vi "map_trap_piastre_stiffback.vi"() -> ()   [LabVIEW 2015]
panel:
  out "Mapping file":string
  in  "Done ?":bool
  in  "KILL":bool
  in  "PAUSE":bool
  in  "RESUME":bool
  in  "QUIT":bool
  in  "Done":bool
  in  "z piastra":bool
  in  "x piastra":bool
  in  "goto y pos":bool
  in  "goto x pos":bool
  in  "End":bool
  in  "zero z - end":bool
  in  "zero x - end":bool
  in  "zero y - end":bool
  in  "positioning done":bool
  out "output":string
  out "command":string
  in  "zero done":bool
  in  "zero z":bool
  in  "zero x":bool
  in  "zero y":bool
  # "Comandi di emergenza"
  # "Posiziono in zero"
  # "Vado sulla piastra \ne azzero"
  # "Vado in posizione\ne parto"
  # "Ritorno a zero"
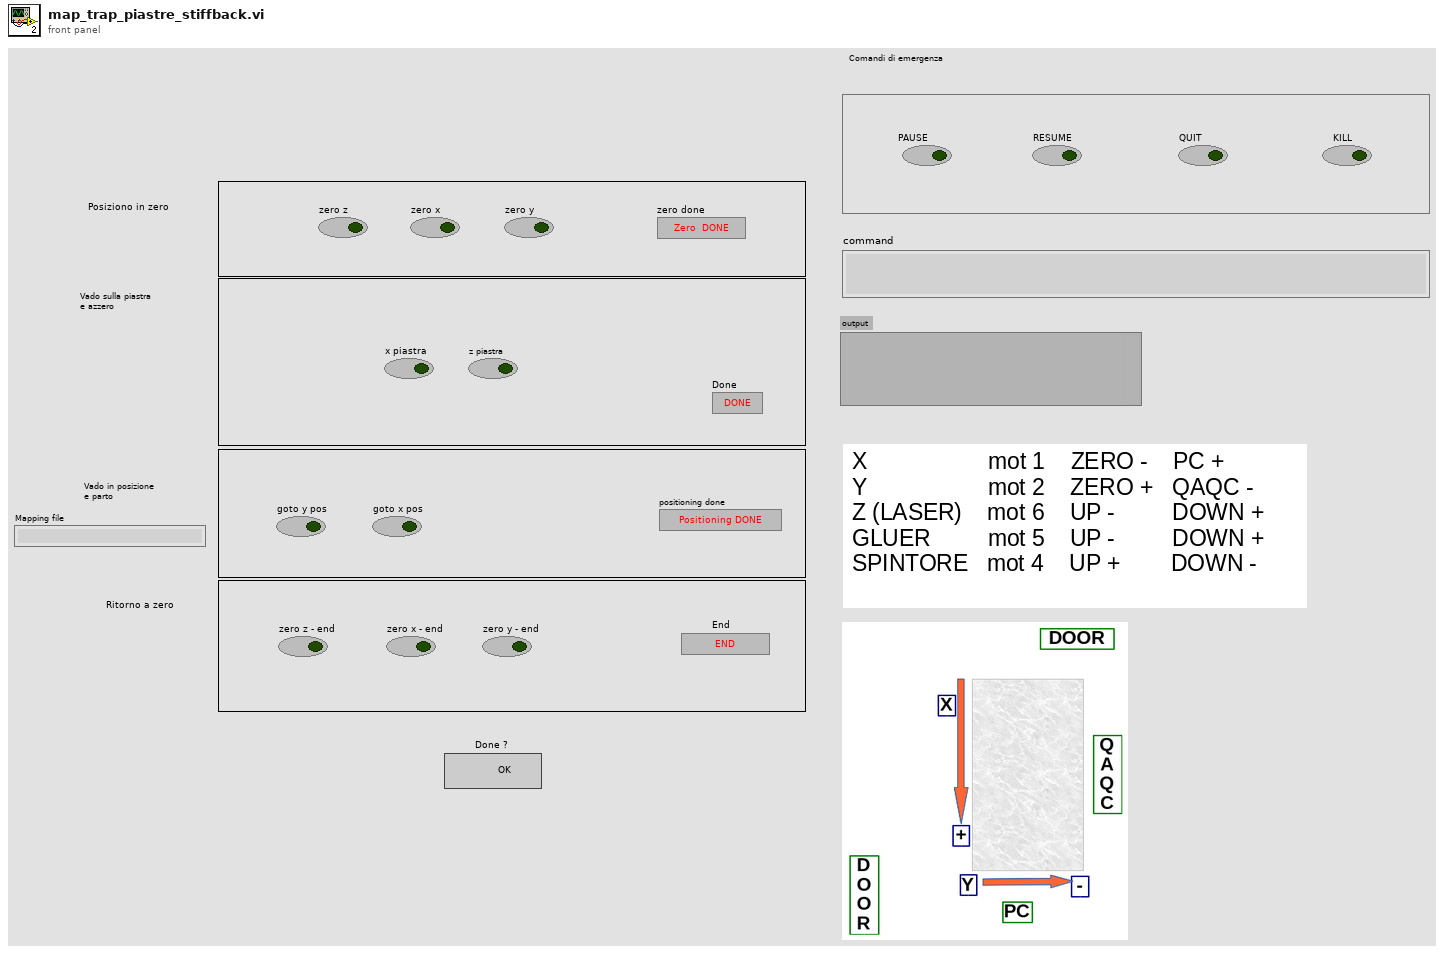
[diagram p1: front panel]
types:
  T1 = enum16{"open", "replace", "create", "open or create", "replace or create", "replace or create with confirmation"}
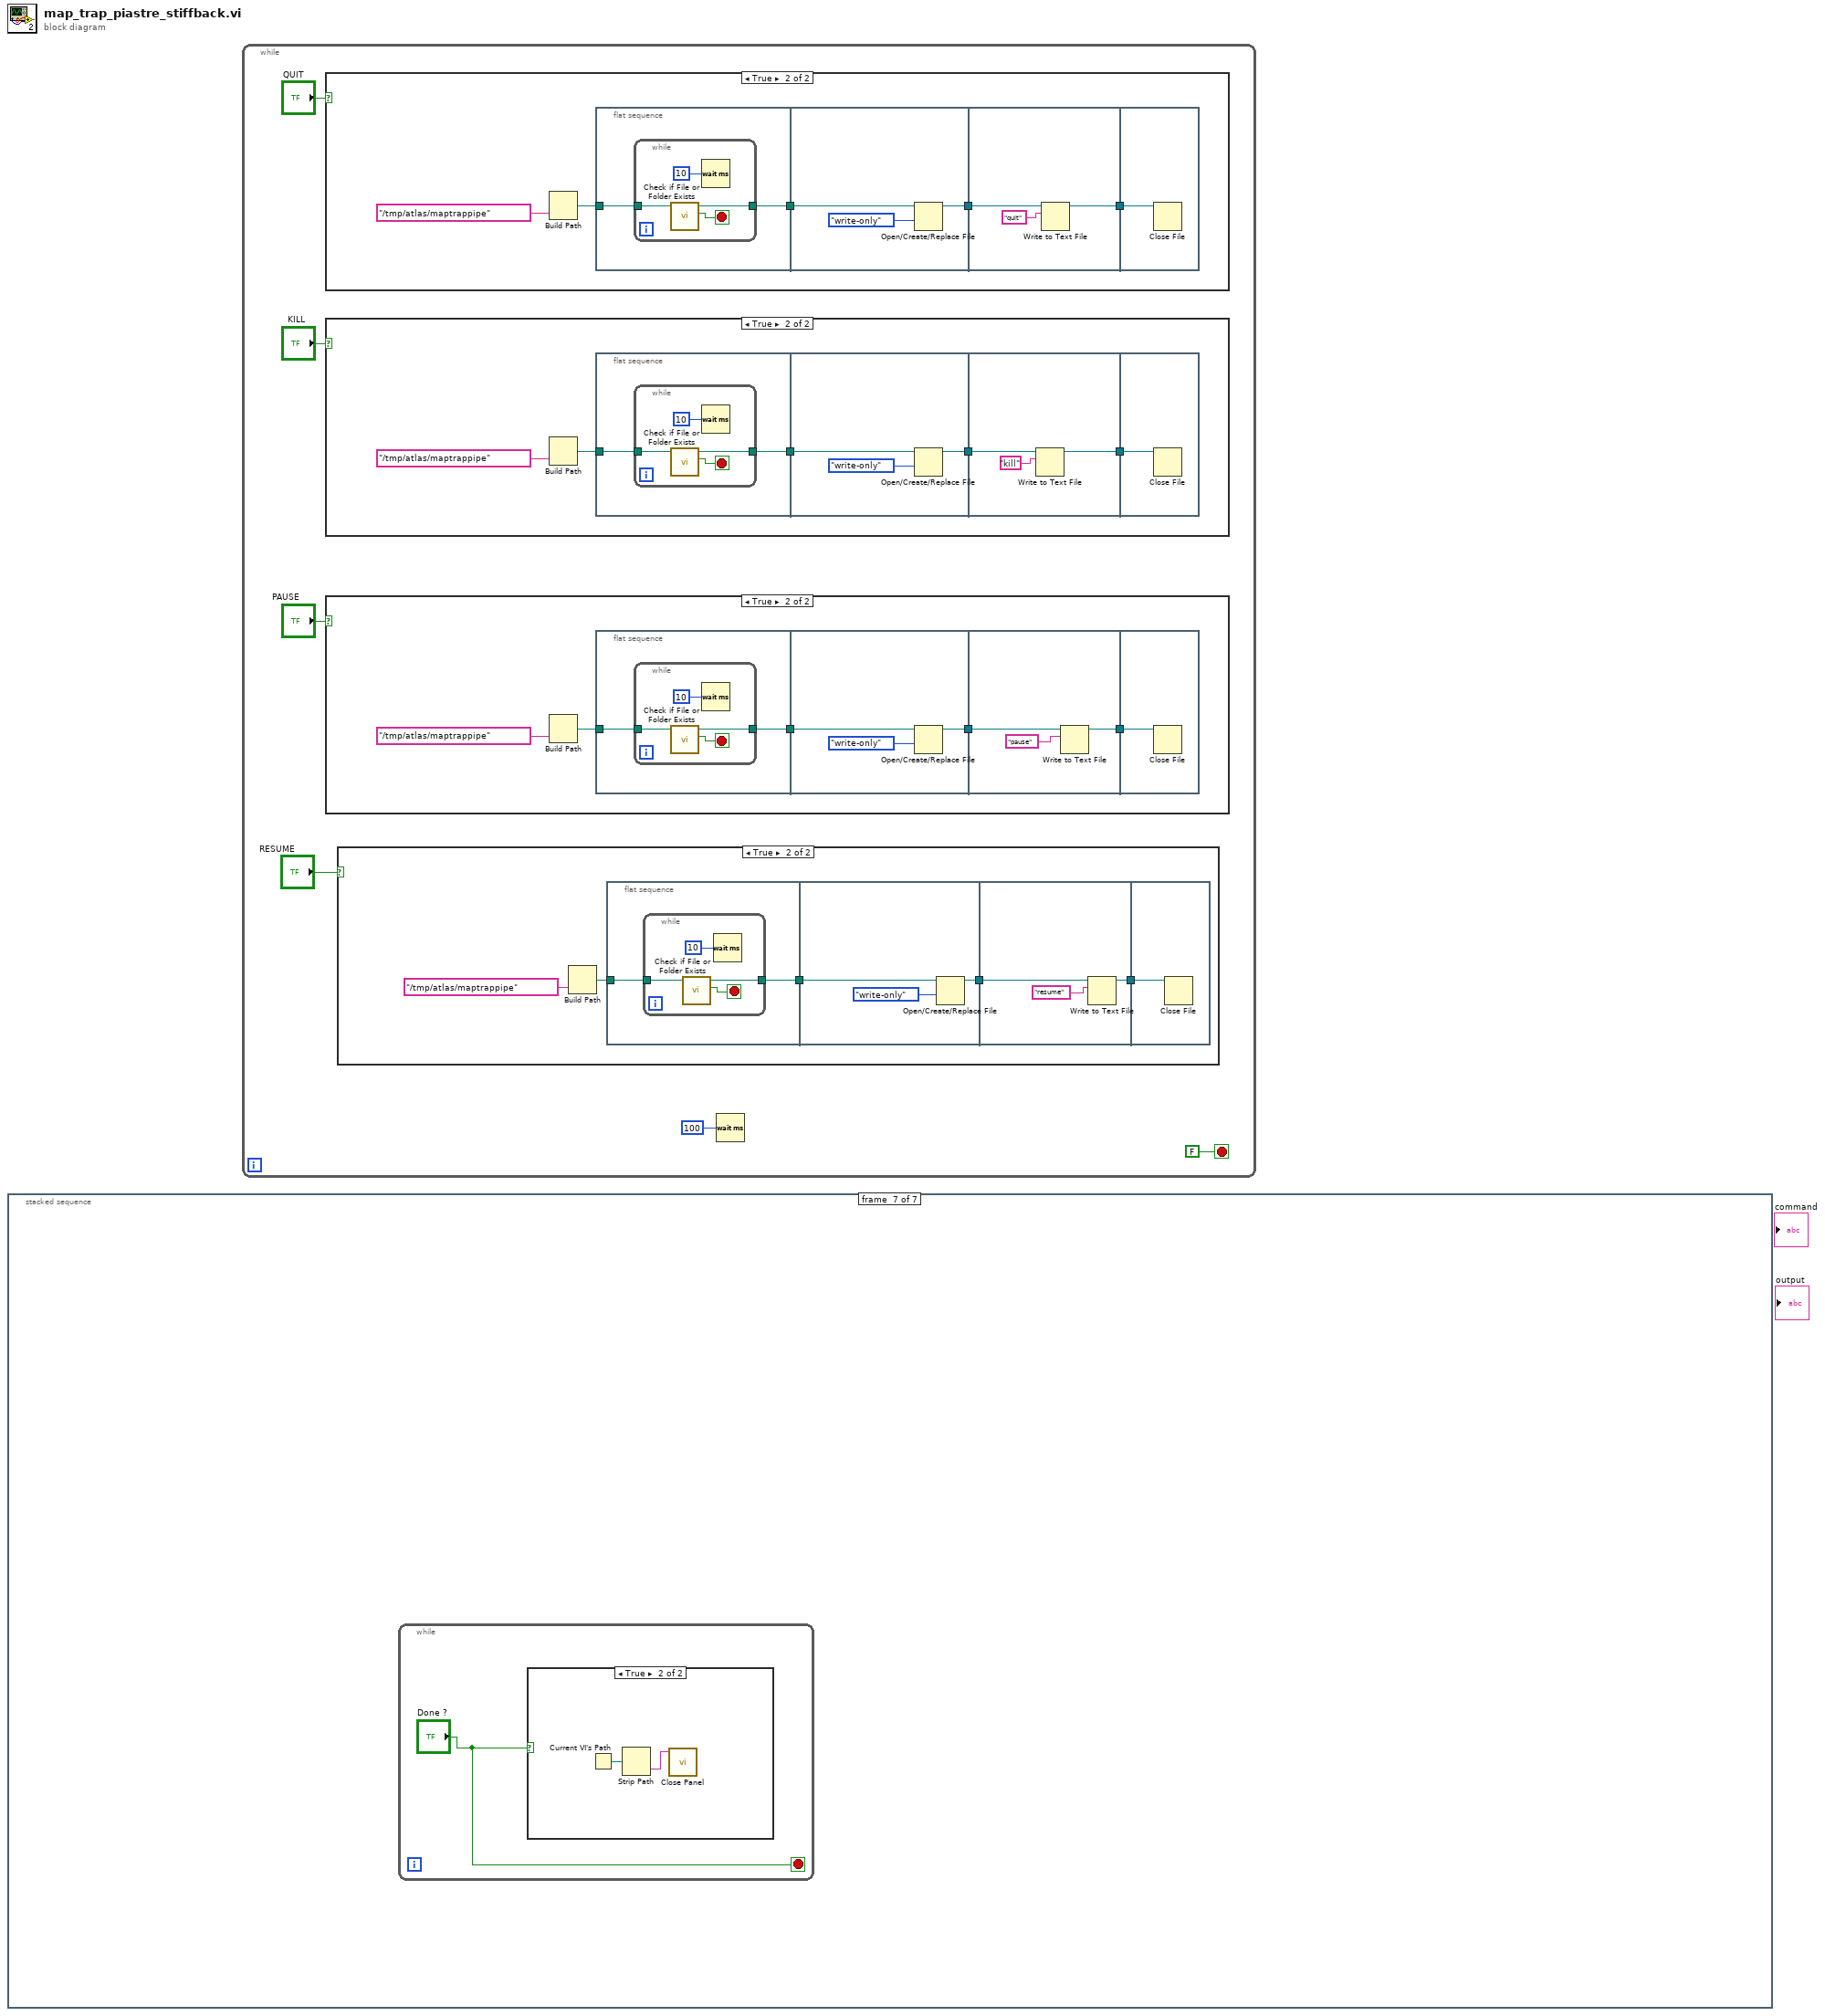
[diagram p0: block diagram]
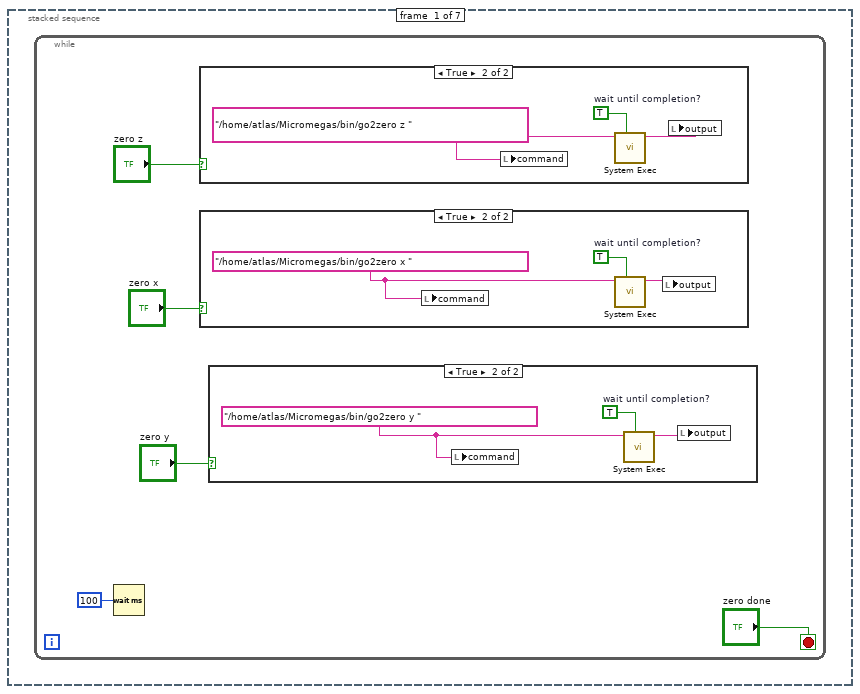
[diagram p6: hidden frame]
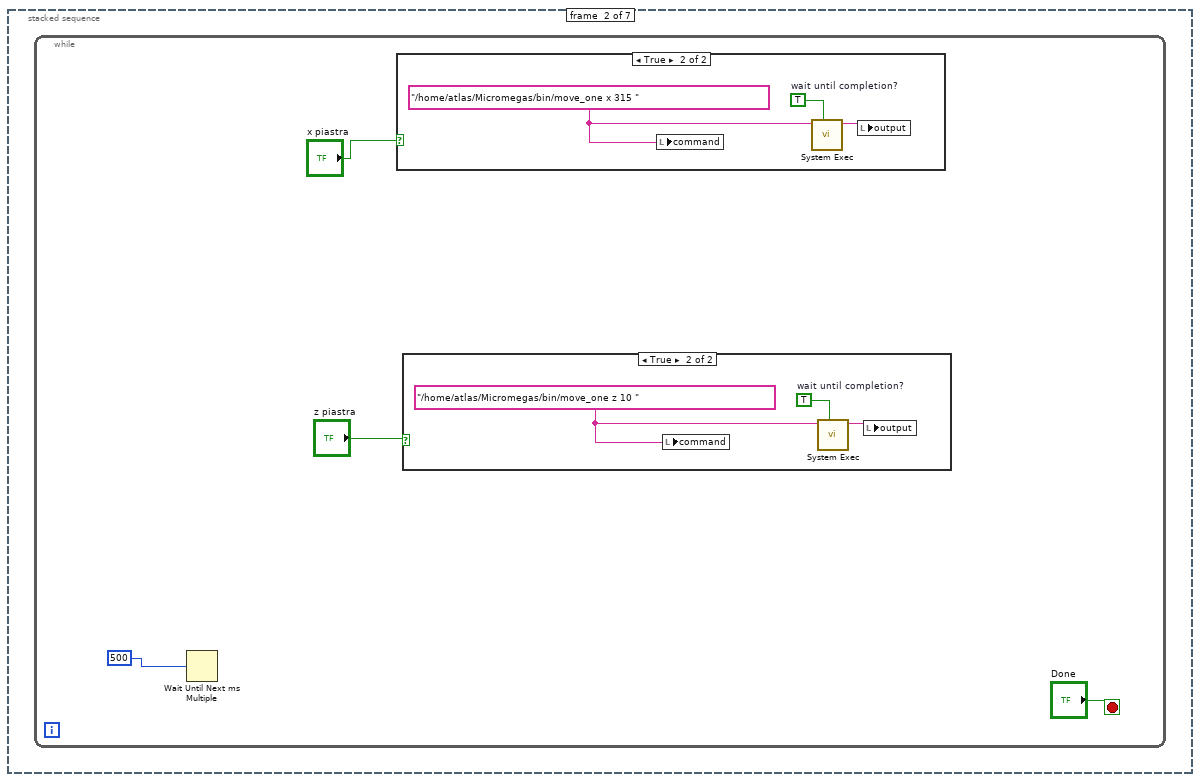
[diagram p10: hidden frame]
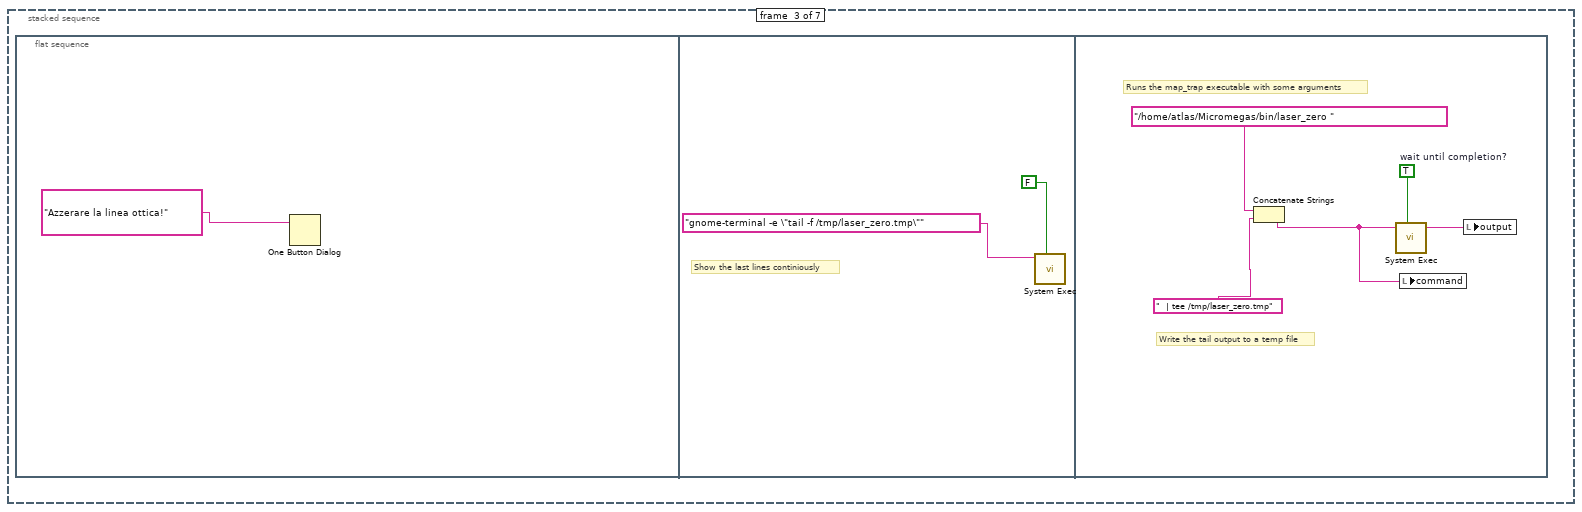
[diagram p13: hidden frame]
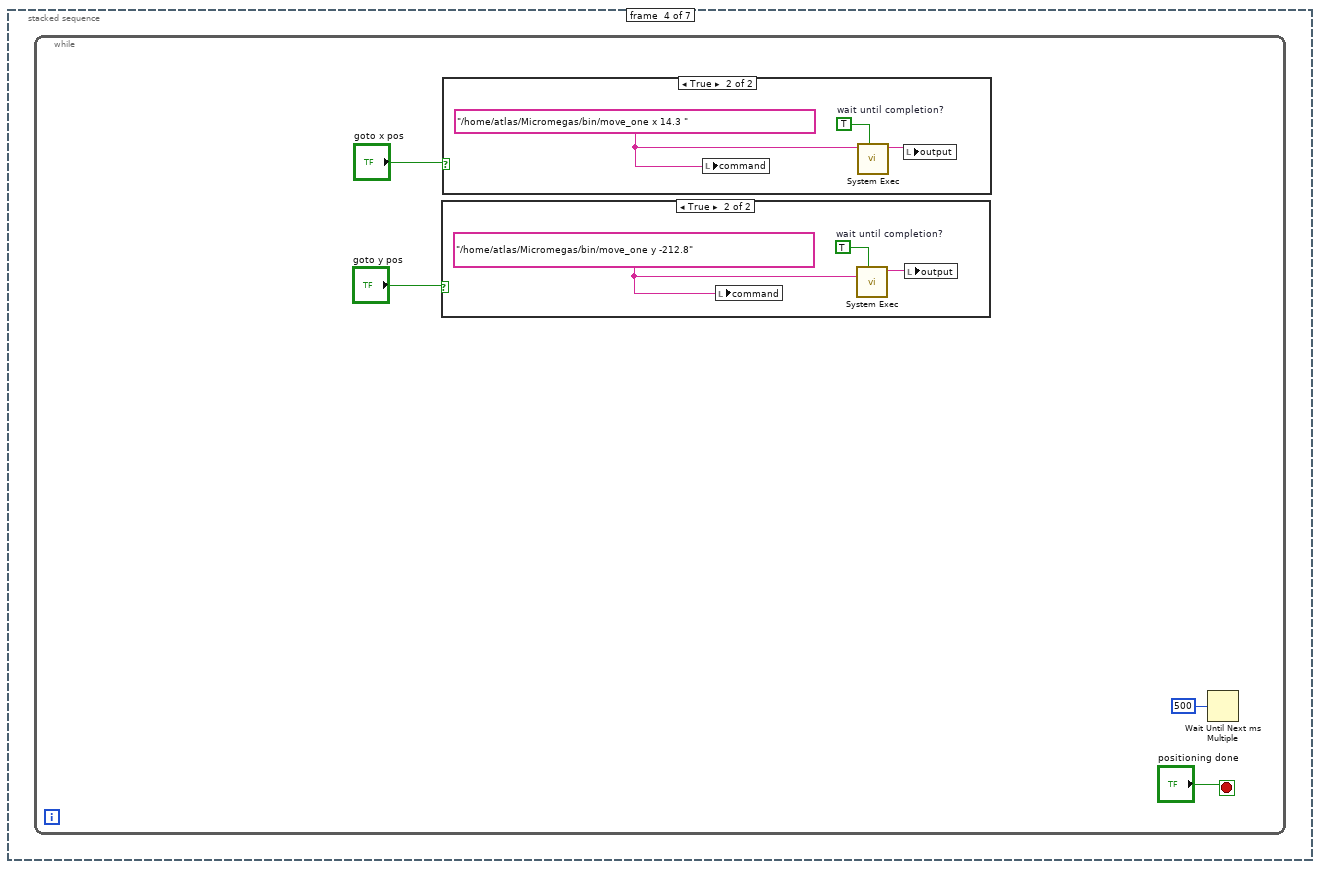
[diagram p14: hidden frame]
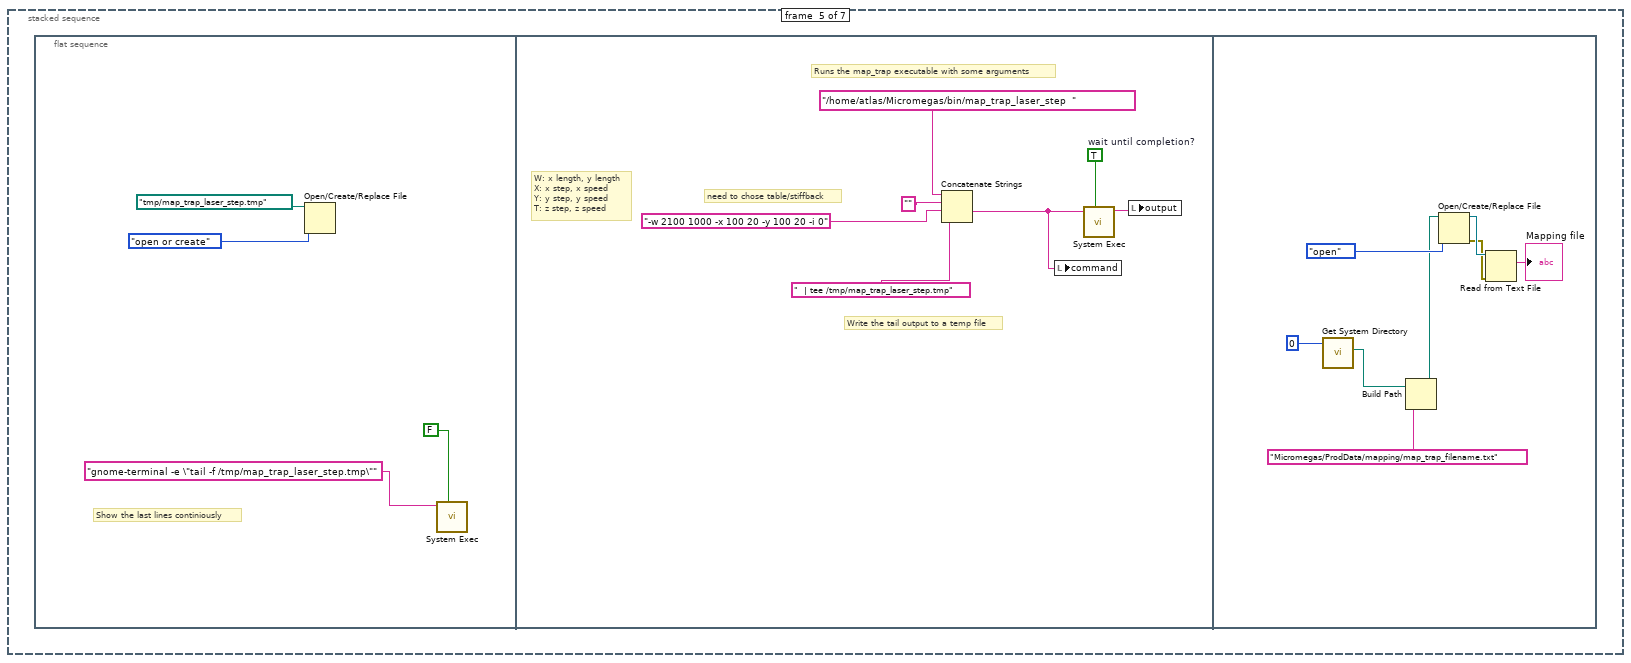
[diagram p17: hidden frame]
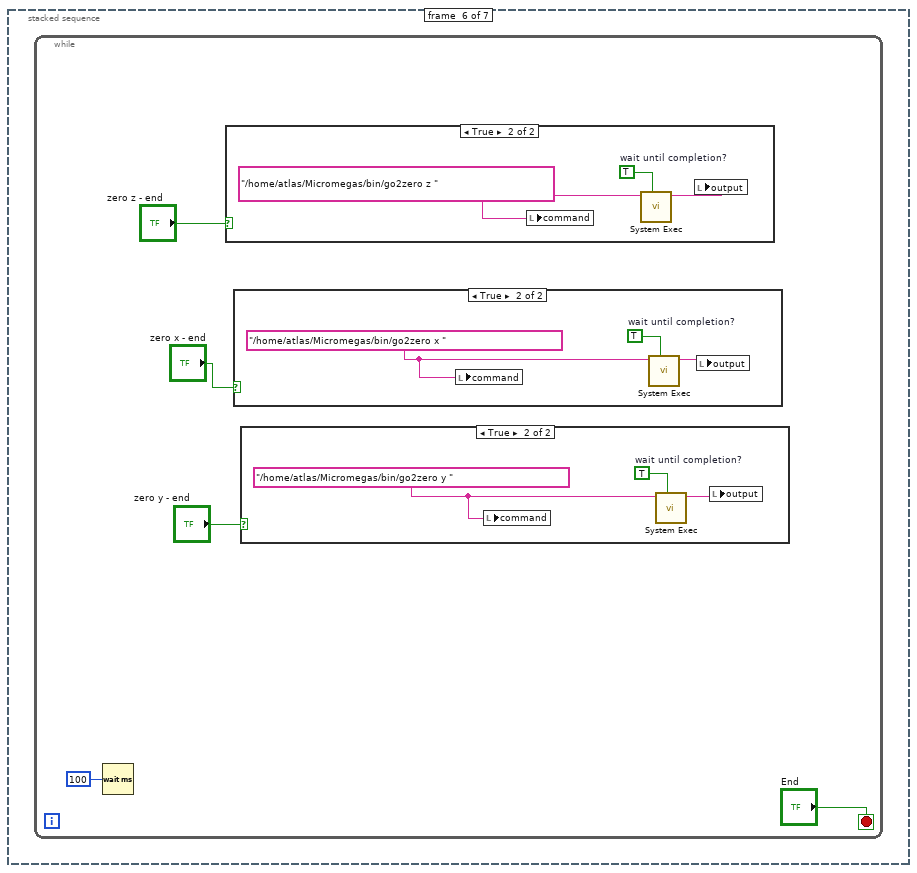
[diagram p18: hidden frame]
diagram:
  n1 = stacked-sequence {
    frame #0 {
      n2 = while {
        stop <- "zero done" stop-if-true
        n3 = Wait (ms)(milliseconds to wait=u32 100) -> ()  [unwired: 1 out]
        n4 = case shown="True" "zero z" {
          frame False {
          }
          frame True {
            w13 = "/home/atlas/Micromegas/bin/go2zero z " ("string")
            w14 = TRUE  # wait until completion?
            n5 = local write "command"(w13) -> ()
            n6 = call <vilib>:"System Exec.vi"("wait until completion? (T)"=w14, "command line"=w13) -> ("standard output"=w12:string)  [unwired: 6 in, 3 out]
            n7 = local write "output"(w12) -> ()
          }
        }
        n8 = case shown="True" "zero x" {
          frame False {
          }
          frame True {
            w10 = "/home/atlas/Micromegas/bin/go2zero x " ("string")
            w11 = TRUE  # wait until completion?
            n9 = local write "command"(w10) -> ()
            n10 = call <vilib>:"System Exec.vi"("wait until completion? (T)"=w11, "command line"=w10) -> ("standard output"=w9:string)  [unwired: 6 in, 3 out]
            n11 = local write "output"(w9) -> ()
          }
        }
        n12 = case shown="True" "zero y" {
          frame False {
          }
          frame True {
            w7 = "/home/atlas/Micromegas/bin/go2zero y " ("string")
            w8 = TRUE  # wait until completion?
            n13 = local write "command"(w7) -> ()
            n14 = call <vilib>:"System Exec.vi"("wait until completion? (T)"=w8, "command line"=w7) -> ("standard output"=w6:string)  [unwired: 6 in, 3 out]
            n15 = local write "output"(w6) -> ()
          }
        }
      }
    }
    frame #1 {
      n16 = while {
        stop <- "Done" stop-if-true
        n17 = Wait Until Next ms Multiple(millisecond multiple=u32 500 ("millisecond timer value")) -> ()  [unwired: 1 out]
        n18 = case shown="True" "x piastra" {
          frame False {
          }
          frame True {
            w22 = "/home/atlas/Micromegas/bin/move_one x 315 " ("string")
            w24 = TRUE  # wait until completion?
            n19 = local write "command"(w22) -> ()
            n20 = call <vilib>:"System Exec.vi"("wait until completion? (T)"=w24, "command line"=w22) -> ("standard output"=w23:string)  [unwired: 6 in, 3 out]
            n21 = local write "output"(w23) -> ()
          }
        }
        n22 = case shown="True" "z piastra" {
          frame False {
          }
          frame True {
            w19 = "/home/atlas/Micromegas/bin/move_one z 10 " ("string")
            w21 = TRUE  # wait until completion?
            n23 = local write "command"(w19) -> ()
            n24 = call <vilib>:"System Exec.vi"("wait until completion? (T)"=w21, "command line"=w19) -> ("standard output"=w20:string)  [unwired: 6 in, 3 out]
            n25 = local write "output"(w20) -> ()
          }
        }
      }
    }
    frame #2 {
      n26 = flat-sequence {
        frame #0 {
          n27 = One Button Dialog(message="Azzerare la linea ottica!") -> ()  [unwired: 1 in, 1 out]
        }
        frame #1 {
          # "Show the last lines continiously"
          n28 = call <vilib>:"System Exec.vi"("wait until completion? (T)"=FALSE, "command line"="gnome-terminal -e \"tail -f /tmp/laser_zero.tmp\"") -> ()  [unwired: 6 in, 4 out]
        }
        frame #2 {
          w32 = TRUE  # wait until completion?
          # "Write the tail output to a temp file"
          # "Runs the map_trap executable with some arguments"
          n29 = Concatenate Strings("/home/atlas/Micromegas/bin/laser_zero " ("string"), "  | tee /tmp/laser_zero.tmp" ("string")) -> (w28:string)
          n30 = call <vilib>:"System Exec.vi"("wait until completion? (T)"=w32, "command line"=w28) -> ("standard output"=w29:string)  [unwired: 6 in, 3 out]
          n31 = local write "command"(w28) -> ()
          n32 = local write "output"(w29) -> ()
        }
      }
    }
    frame #3 {
      n33 = while {
        stop <- "positioning done" stop-if-true
        n34 = case shown="True" "goto y pos" {
          frame False {
          }
          frame True {
            w37 = "/home/atlas/Micromegas/bin/move_one y -212.8" ("string")
            w39 = TRUE  # wait until completion?
            n35 = local write "command"(w37) -> ()
            n36 = call <vilib>:"System Exec.vi"("wait until completion? (T)"=w39, "command line"=w37) -> ("standard output"=w38:string)  [unwired: 6 in, 3 out]
            n37 = local write "output"(w38) -> ()
          }
        }
        n38 = case shown="True" "goto x pos" {
          frame False {
          }
          frame True {
            w40 = "/home/atlas/Micromegas/bin/move_one x 14.3 " ("string")
            w42 = TRUE  # wait until completion?
            n39 = local write "command"(w40) -> ()
            n40 = call <vilib>:"System Exec.vi"("wait until completion? (T)"=w42, "command line"=w40) -> ("standard output"=w41:string)  [unwired: 6 in, 3 out]
            n41 = local write "output"(w41) -> ()
          }
        }
        n42 = Wait Until Next ms Multiple(millisecond multiple=u32 500) -> ()  [unwired: 1 out]
      }
    }
    frame #4 {
      n43 = flat-sequence {
        frame #0 {
          # "Show the last lines continiously"
          n44 = Open/Create/Replace File(file path (use dialog)=path "/tmp/map_trap_laser_step.tmp", operation (0:open)=T1."open or create") -> ()  [unwired: 4 in, 3 out]
          n45 = call <vilib>:"System Exec.vi"("wait until completion? (T)"=FALSE, "command line"="gnome-terminal -e \"tail -f /tmp/map_trap_laser_step.tmp\"") -> ()  [unwired: 6 in, 4 out]
        }
        frame #1 {
          w53 = TRUE  # wait until completion?
          # "need to chose table/stiffback"
          # "Write the tail output to a temp file"
          # "Runs the map_trap executable with some arguments"
          # "W: x length, y length\nX: x step, x speed\nY: y step, y speed\nT: z step, z speed"
          n46 = Concatenate Strings("/home/atlas/Micromegas/bin/map_trap_laser_step  " ("string"), "" ("string"), "-w 2100 1000 -x 100 20 -y 100 20 -i 0" ("string"), "  | tee /tmp/map_trap_laser_step.tmp" ("string")) -> (w48:string)
          n47 = local write "command"(w48) -> ()
          n48 = call <vilib>:"System Exec.vi"("wait until completion? (T)"=w53, "command line"=w48) -> ("standard output"=w47:string)  [unwired: 6 in, 3 out]
          n49 = local write "output"(w47) -> ()
        }
        frame #2 {
          n50 = call <vilib>:"Get System Directory.vi"("system directory type"=0) -> ("system directory"=w55:path)  [unwired: 10 in]
          n51 = Build Path(base path=w55, name or relative path="Micromegas/ProdData/mapping/map_trap_filename.txt") -> (appended path=w54:path)
          n52 = Open/Create/Replace File(file path (use dialog)=w54, operation (0:open)=T1."open") -> (refnum out=w60:refnum<file>, error out=w59:errorcluster)  [unwired: 4 in, 1 out]
          n53 = Read from Text File(file (use dialog)=w60, error in=w59) -> (text=→"Mapping file":string)  [unwired: 2 in, 3 out]
        }
      }
    }
    frame #5 {
      n54 = while {
        stop <- "End" stop-if-true
        n55 = Wait (ms)(milliseconds to wait=u32 100) -> ()  [unwired: 1 out]
        n56 = case shown="True" "zero z - end" {
          frame False {
          }
          frame True {
            w74 = "/home/atlas/Micromegas/bin/go2zero z " ("string")
            w75 = TRUE  # wait until completion?
            n57 = local write "command"(w74) -> ()
            n58 = call <vilib>:"System Exec.vi"("wait until completion? (T)"=w75, "command line"=w74) -> ("standard output"=w73:string)  [unwired: 6 in, 3 out]
            n59 = local write "output"(w73) -> ()
          }
        }
        n60 = case shown="True" "zero x - end" {
          frame False {
          }
          frame True {
            w71 = "/home/atlas/Micromegas/bin/go2zero x " ("string")
            w72 = TRUE  # wait until completion?
            n61 = local write "command"(w71) -> ()
            n62 = call <vilib>:"System Exec.vi"("wait until completion? (T)"=w72, "command line"=w71) -> ("standard output"=w70:string)  [unwired: 6 in, 3 out]
            n63 = local write "output"(w70) -> ()
          }
        }
        n64 = case shown="True" "zero y - end" {
          frame False {
          }
          frame True {
            w68 = "/home/atlas/Micromegas/bin/go2zero y " ("string")
            w69 = TRUE  # wait until completion?
            n65 = local write "command"(w68) -> ()
            n66 = call <vilib>:"System Exec.vi"("wait until completion? (T)"=w69, "command line"=w68) -> ("standard output"=w67:string)  [unwired: 6 in, 3 out]
            n67 = local write "output"(w67) -> ()
          }
        }
      }
    }
    frame #6 {
      n68 = while {
        stop <- "Done ?" stop-if-true
        n69 = case shown="True" "Done ?" {
          frame False {
          }
          frame True {
            n70 = Current VI's Path() -> (path=w77:path)
            n71 = Strip Path(path=w77) -> (name=w78:string)  [unwired: 1 out]
            n72 = call <vilib>:"Close Panel.vi"("VI name"=w78) -> ()  [unwired: 10 in, 1 out]
          }
        }
      }
    }
  }
  n73 = while {
    stop <- FALSE stop-if-true
    n74 = case shown="True" "QUIT" {
      frame False {
      }
      frame True {
        n75 = Build Path(name or relative path="/tmp/atlas/maptrappipe" ("string")) -> (appended path=w139:path)  [unwired: 1 in]
        n76 = flat-sequence {
          tunnel: [w145] -> w143
          tunnel: w139 -> [w144]
          tunnel: w143 -> [w152]
          tunnel: [w150] -> w142
          tunnel: w142 -> [w155]
          tunnel: [w154] -> w141
          tunnel: w141 -> [w156]
          frame #0 {
            n77 = while {
              tunnel: [w147] -> w145
              tunnel: w144 -> [w146]
              stop <- w148 stop-if-true
              n78 = call <vilib>:"Check if File or Folder Exists.vi"("path"=w146) -> ("file or folder exists?"=w148:bool, "dup path"=w147:path)  [unwired: 8 in, 1 out]
              n79 = Wait (ms)(milliseconds to wait=u32 10) -> ()  [unwired: 1 out]
            }
          }
          frame #1 {
            n80 = Open/Create/Replace File(file path (use dialog)=w152, access (0:read/write)=enum16{"read/write", "read-only", "write-only"}."write-only") -> (refnum out=w150:refnum<file>)  [unwired: 4 in, 2 out]
          }
          frame #2 {
            n81 = Write to Text File(file (use dialog)=w155, text="quit") -> (refnum out=w154:refnum<file>)  [unwired: 2 in, 2 out]
          }
          frame #3 {
            n82 = Close File(refnum=w156) -> ()  [unwired: 1 in, 2 out]
          }
        }
      }
    }
    n83 = case shown="True" "KILL" {
      frame False {
      }
      frame True {
        n84 = Build Path(name or relative path="/tmp/atlas/maptrappipe" ("string")) -> (appended path=w103:path)  [unwired: 1 in]
        n85 = flat-sequence {
          tunnel: [w109] -> w107
          tunnel: w103 -> [w108]
          tunnel: w107 -> [w116]
          tunnel: [w114] -> w106
          tunnel: w106 -> [w119]
          tunnel: [w118] -> w105
          tunnel: w105 -> [w120]
          frame #0 {
            n86 = while {
              tunnel: [w111] -> w109
              tunnel: w108 -> [w110]
              stop <- w112 stop-if-true
              n87 = call <vilib>:"Check if File or Folder Exists.vi"("path"=w110) -> ("file or folder exists?"=w112:bool, "dup path"=w111:path)  [unwired: 8 in, 1 out]
              n88 = Wait (ms)(milliseconds to wait=u32 10) -> ()  [unwired: 1 out]
            }
          }
          frame #1 {
            n89 = Open/Create/Replace File(file path (use dialog)=w116, access (0:read/write)=enum16{"read/write", "read-only", "write-only"}."write-only") -> (refnum out=w114:refnum<file>)  [unwired: 4 in, 2 out]
          }
          frame #2 {
            n90 = Write to Text File(file (use dialog)=w119, text="kill") -> (refnum out=w118:refnum<file>)  [unwired: 2 in, 2 out]
          }
          frame #3 {
            n91 = Close File(refnum=w120) -> ()  [unwired: 1 in, 2 out]
          }
        }
      }
    }
    n92 = case shown="True" "PAUSE" {
      frame False {
      }
      frame True {
        n93 = Build Path(name or relative path="/tmp/atlas/maptrappipe" ("string")) -> (appended path=w85:path)  [unwired: 1 in]
        n94 = flat-sequence {
          tunnel: [w91] -> w89
          tunnel: w85 -> [w90]
          tunnel: w89 -> [w98]
          tunnel: [w96] -> w88
          tunnel: w88 -> [w101]
          tunnel: [w100] -> w87
          tunnel: w87 -> [w102]
          frame #0 {
            n95 = while {
              tunnel: [w93] -> w91
              tunnel: w90 -> [w92]
              stop <- w94 stop-if-true
              n96 = call <vilib>:"Check if File or Folder Exists.vi"("path"=w92) -> ("file or folder exists?"=w94:bool, "dup path"=w93:path)  [unwired: 8 in, 1 out]
              n97 = Wait (ms)(milliseconds to wait=u32 10) -> ()  [unwired: 1 out]
            }
          }
          frame #1 {
            n98 = Open/Create/Replace File(file path (use dialog)=w98, access (0:read/write)=enum16{"read/write", "read-only", "write-only"}."write-only") -> (refnum out=w96:refnum<file>)  [unwired: 4 in, 2 out]
          }
          frame #2 {
            n99 = Write to Text File(file (use dialog)=w101, text="pause") -> (refnum out=w100:refnum<file>)  [unwired: 2 in, 2 out]
          }
          frame #3 {
            n100 = Close File(refnum=w102) -> ()  [unwired: 1 in, 2 out]
          }
        }
      }
    }
    n101 = case shown="True" "RESUME" {
      frame False {
      }
      frame True {
        n102 = Build Path(name or relative path="/tmp/atlas/maptrappipe" ("string")) -> (appended path=w121:path)  [unwired: 1 in]
        n103 = flat-sequence {
          tunnel: [w127] -> w125
          tunnel: w121 -> [w126]
          tunnel: w125 -> [w134]
          tunnel: [w132] -> w124
          tunnel: w124 -> [w137]
          tunnel: [w136] -> w123
          tunnel: w123 -> [w138]
          frame #0 {
            n104 = while {
              tunnel: [w129] -> w127
              tunnel: w126 -> [w128]
              stop <- w130 stop-if-true
              n105 = call <vilib>:"Check if File or Folder Exists.vi"("path"=w128) -> ("file or folder exists?"=w130:bool, "dup path"=w129:path)  [unwired: 8 in, 1 out]
              n106 = Wait (ms)(milliseconds to wait=u32 10) -> ()  [unwired: 1 out]
            }
          }
          frame #1 {
            n107 = Open/Create/Replace File(file path (use dialog)=w134, access (0:read/write)=enum16{"read/write", "read-only", "write-only"}."write-only") -> (refnum out=w132:refnum<file>)  [unwired: 4 in, 2 out]
          }
          frame #2 {
            n108 = Write to Text File(file (use dialog)=w137, text="resume") -> (refnum out=w136:refnum<file>)  [unwired: 2 in, 2 out]
          }
          frame #3 {
            n109 = Close File(refnum=w138) -> ()  [unwired: 1 in, 2 out]
          }
        }
      }
    }
    n110 = Wait (ms)(milliseconds to wait=100) -> ()  [unwired: 1 out]
  }
